vi "Motion blur (subVI).vi"(8 "Y":dbl[](array[numeric]), 10 "pixel size [um]":dbl, 11 "waist radius [um]":dbl) -> (2 "N":i32, 3 "output":dbl[](array[numeric]))   [LabVIEW 2024]
uses:
  <vilib>/Analysis/2dsp.llb/1D Convolution (DBL).vi
  <vilib>/Analysis/NI_AALPro.lvlib
panel:
  out "Array":dbl[](array[numeric])
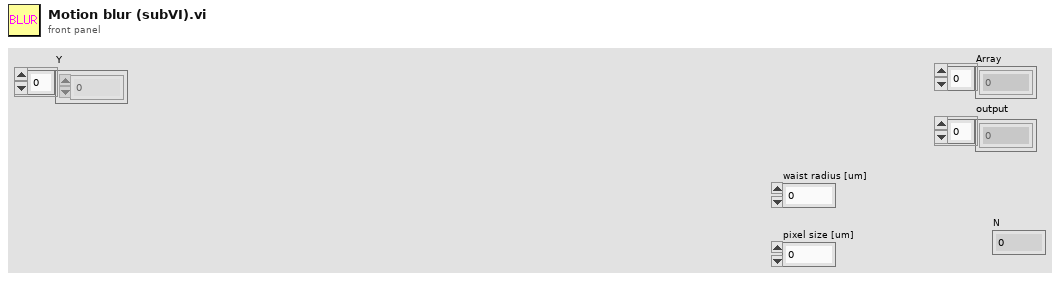
[diagram p1: front panel]
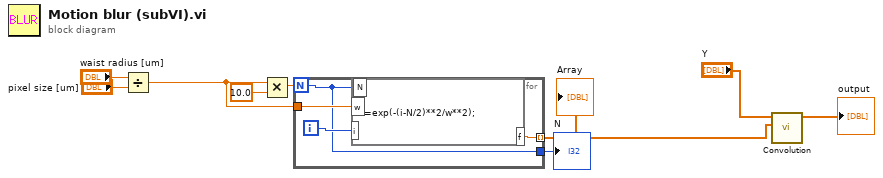
[diagram p0: block diagram]
diagram:
  n1 = Divide(x="waist radius [um]", y="pixel size [um]") -> (x/y=w5:dbl)
  n2 = Multiply(x=w5, y=10.0) -> (x*y=w6:dbl)
  n3 = for {
    N: w6 -> [w10]
    tunnel: [w12] -> w2 mode=indexing
    tunnel: w5 -> [w11]
    tunnel: [w10] -> w4
    i -> [w13]
    n4 = formula code="f=exp(-(i-N/2)**2/w**2);"("i"=w13, "N"=w10, "w"=w11) -> ("f"=w12:dbl)
  }
  "Array" <- w2
  "N" <- w4
  n5 = call-poly <vilib>:"Convolution.vi"("Y"=w2, "X"="Y") -> ("X * Y"=→"output":dbl[])  [unwired: 8 in, 1 out]
